vi "Handle Error.vi"(8 "error in (no error)":errorcluster, 11 "MSS Remote Actor in":refnum<class "MSS Remote Actor.lvclass">) -> (0 "error out":errorcluster, 2 "stop actor?":bool=TRUE, 3 "MSS Remote Actor out":refnum<class "MSS Remote Actor.lvclass">)   [LabVIEW 2023]
doc: "(<B>Filename</B>: Actor Framework.lvlib:Actor.lvclass:Handle Error.vi)\n\nDefines how the actor handles an error that occurred while processing a message. By default, this method does nothing except stop the actor."
uses:
  MSS Remote Actor.lvclass
  AF Helpers/My Actor/My Actor/My Actor.lvclass
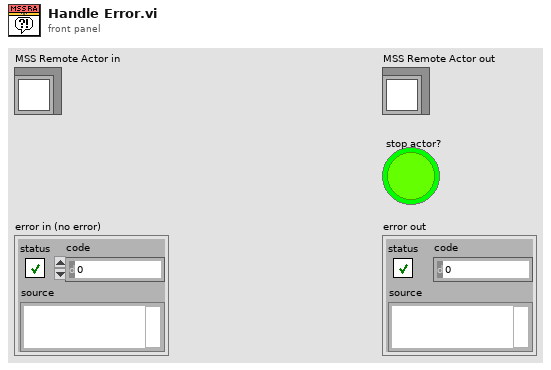
[diagram p1: front panel]
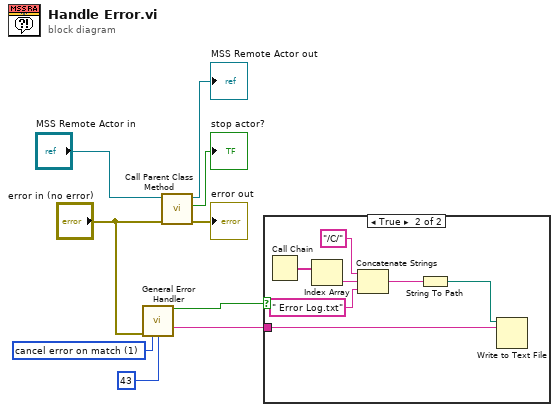
[diagram p0: block diagram]
diagram:
  w5 = 1 items=["no exception", "cancel error on match", "set error on match"] ("[exception action] (none:0)")
  n1 = call <vilib>:"General Error Handler.vi"("error in (no error)"="error in (no error)", "[exception action] (none:0)"=w5, "[exception code]"=43) -> ("error?"=w1:bool, "message"=w2:string)  [unwired: 8 in, 3 out]
  n2 = call-parent "Call Parent Class Method"("error in (no error)"="error in (no error)", "Actor in"="MSS Remote Actor in") -> ("error out"=→"error out":errorcluster, "stop actor?"=→"stop actor?":bool, "Actor out"=→"MSS Remote Actor out":refnum<class "MSS Remote Actor.lvclass">)  [unwired: 7 in]
  n3 = case shown="True" w1 {
    tunnel: w2 -> [_ w10]
    frame False {
    }
    frame True {
      n4 = Call Chain() -> (call chain=w16:string[])
      n5 = Index Array(array=w16) -> (element=w15:string)  [unwired: 1 in]
      n6 = Concatenate Strings("/C/" ("string"), w15, " Error Log.txt" ("string")) -> (w12:string)
      n7 = String To Path(string=w12) -> (path=w11:path)
      n8 = Write to Text File(file (use dialog)=w11, text=w10) -> ()  [unwired: 2 in, 3 out]
    }
  }
